vi "if VI is idle run VI.vi"(8 "error in (no error)":errorcluster, 11 "VI in":refnum<vi>) -> (0 "error out":errorcluster, 3 "VI out":refnum<vi>)   [LabVIEW 2023]
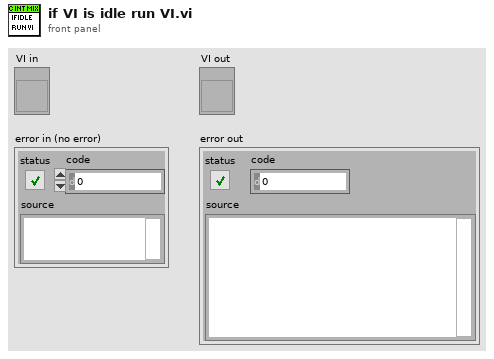
[diagram p1: front panel]
types:
  T1 = enum32{"Bad", "Idle", "Run top level", "Running"}
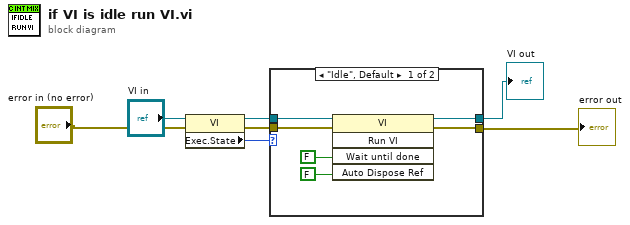
[diagram p0: block diagram]
diagram:
  n1 = property class="VI"(reference="VI in", error in="error in (no error)") -> (reference out=w5:refnum<vi>, error out=w4:errorcluster, "Exec.State"=w3:T1)
  n2 = case shown="\"Idle\", Default" w3 {
    tunnel: w4 -> [w9 w14]
    tunnel: w5 -> [w11 w15]
    tunnel: [w10 w15] -> w6
    tunnel: [w8 w14] -> w7
    frame "Idle", Default {
      n3 = invoke class="VI" method="Run VI"(reference=w11, error in=w9, "Wait until done"=FALSE ("Wait Until Done"), "Auto Dispose Ref"=FALSE ("Auto Dispose Reference")) -> (reference out=w10:refnum<vi>, error out=w8:errorcluster)  [unwired: 1 in, 3 out]
    }
    frame "Run top level", "Running" {
    }
  }
  "error out" <- w7
  "VI out" <- w6
